vi "createAxisString.vi"(10 "PlotsString":string, 11 "Input Data":T1) -> (3 "AxisString":string)   [LabVIEW 2012]
uses:
  pgfPlotAxis_tdef.ctl
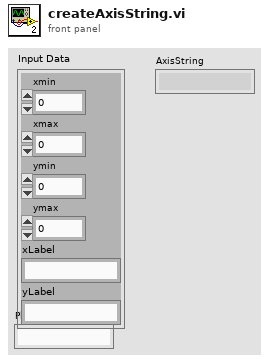
[diagram p1: front panel]
types:
  T1 = typedef "pgfPlotAxis_tdef.ctl" = cluster{"xmin":dbl, "xmax":dbl, "ymin":dbl, "ymax":dbl, "xLabel":string, "yLabel":string}
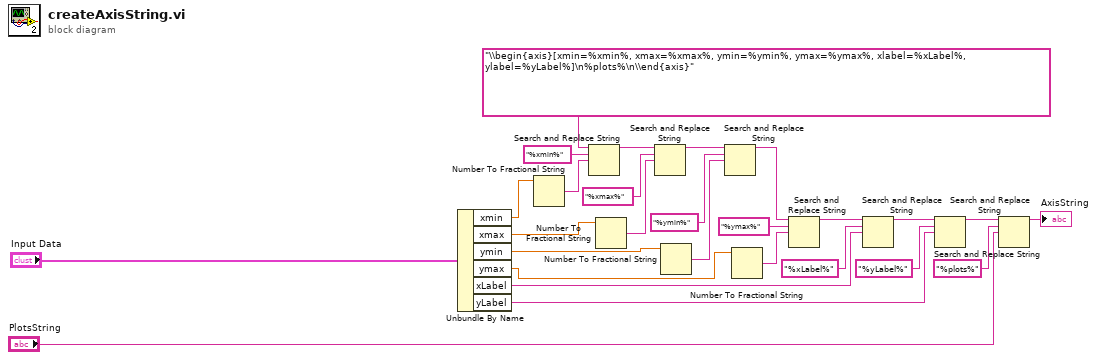
[diagram p0: block diagram]
diagram:
  n1 = Unbundle By Name("Input Data") -> ("xmin"=w18:dbl, "xmax"=w19:dbl, "ymin"=w20:dbl, "ymax"=w21:dbl, "xLabel"=w22:string, "yLabel"=w23:string)
  n2 = Number To Fractional String(number=w18) -> (F-format string=w10:string)  [unwired: 3 in]
  n3 = Search and Replace String(input string="\\begin{axis}[xmin=%xmin%, xmax=%xmax%, ymin=%ymin%, ymax=%ymax%, xlabel=%xLabel%, ylabel=%yLabel%]\n%plots%\n\\end{axis}", search string="%xmin%", replace string=w10) -> (result string=w3:string)  [unwired: 5 in, 3 out]
  n4 = Number To Fractional String(number=w19) -> (F-format string=w9:string)  [unwired: 3 in]
  n5 = Search and Replace String(input string=w3, search string="%xmax%", replace string=w9) -> (result string=w2:string)  [unwired: 5 in, 3 out]
  n6 = Number To Fractional String(number=w20) -> (F-format string=w6:string)  [unwired: 3 in]
  n7 = Search and Replace String(input string=w2, search string="%ymin%", replace string=w6) -> (result string=w1:string)  [unwired: 5 in, 3 out]
  n8 = Number To Fractional String(number=w21) -> (F-format string=w5:string)  [unwired: 3 in]
  n9 = Search and Replace String(input string=w1, search string="%ymax%", replace string=w5) -> (result string=w16:string)  [unwired: 5 in, 3 out]
  n10 = Search and Replace String(input string=w16, search string="%xLabel%", replace string=w22) -> (result string=w12:string)  [unwired: 5 in, 3 out]
  n11 = Search and Replace String(input string=w12, search string="%yLabel%", replace string=w23) -> (result string=w25:string)  [unwired: 5 in, 3 out]
  n12 = Search and Replace String(input string=w25, search string="%plots%", replace string="PlotsString") -> (result string=→"AxisString":string)  [unwired: 5 in, 3 out]
